vi "niFPGALMRsmpl1MOutSCTL.vi"(0 "input data":fxp<+/-,16,1>, 1 "reset":bool) -> (3 "channel index":u8, 4 "output data":fxp<+/-,18,1> format="%.18g", 10 "output valid":bool)   [LabVIEW 2017]
uses:
  <vilib>/Platform/TimedLoop/XDataNode/timing_clust.ctl
  <vilib>/Platform/TimedLoop/XDataNode/nitl_modes.ctl
  <vilib>/Platform/TimedLoop/XDataNode/wakeup.ctl
  <vilib>/Platform/TimedLoop/XDataNode/XDataNode.xnode
  <vilib>/Platform/TimedLoop/XDataNode/XDNodeRunTimeDep.lvlib
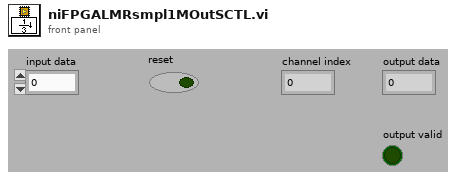
[diagram p1: front panel]
types:
  T1 = typedef "XDNodeRunTimeDep.lvlib/timing_clust.ctl" = cluster{"Expected End [f-1]":u64, "Actual End [f-1]":u64, "Finished Late? [f-1]":bool, "Expected End [i-1]":u64, "Actual End [i-1]":u64, "Finished Late? [i-1]":bool, "Expected Start [i]":u64, "Actual Start [i]":u64, "Expected Start [f]":u64, "Actual Start [f]":u64, "Source Name":string, "Structure Name":string, "Period":i64, "Deadline":i64, "Offset":i64, "Start":i64, "Priority":i32, "Timeout":i32, "Mode":T2, "Wakeup Reason":T3, "Error":errorcluster, "Source Type":string, "Secondary Source Type":string, "Global End Time":u64, "Global Start Time":u64, "Frame Duration":u64, "Iteration Duration":u64, "Assigned CPU":i32, "I/O Scan Engine Mode":u32}
  T2 = typedef "XDNodeRunTimeDep.lvlib/nitl_modes.ctl" = enum32{"No Change", "Process missed periods, maintain original phase", "Discard missed periods, maintain original phase", "Process missed periods, ignore original phase", "Discard missed periods, ignore original phase"}
  T3 = typedef "XDNodeRunTimeDep.lvlib/wakeup.ctl" = enum32{"Normal", "Aborted", "Asynchronous wakeup", "Timing source error", "Timed loop error", "Timeout"}
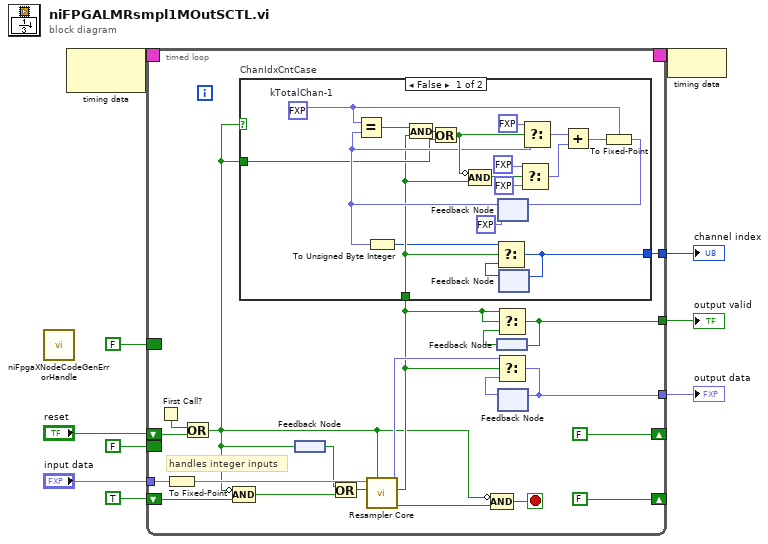
[diagram p0: block diagram]
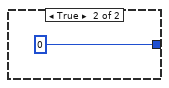
[diagram p2: hidden frame]
diagram:
  n1 = call <vilib>:"niFpgaXNodeCodeGenErrorHandle.vi"() -> ()  [unwired: 1 in]
  n2 = node-c288 ("Input Node")() -> (w8:T1)  [unwired: 1 out]
  n3 = timed-loop "Timed Loop" {
    timing: w8 -> [_]
    timing-out: [_] -> w7
    tunnel: "input data" -> [w27]
    tunnel: [w21] -> w9
    tunnel: [w23] -> w10
    border: FALSE ("dataReady?") -> [_]
    shift-right: [FALSE] -> _
    shift-left: "reset" -> [w17]
    tunnel: [w18] -> w5
    shift-right: [FALSE] -> _
    shift-left: TRUE -> [w25]
    border: FALSE ("reset") -> [_]
    stop <- w22 stop-if-true
    # "handles integer inputs"
    n4 = First Call?() -> (First Call?: T/F=w16:bool)
    n5 = To Fixed-Point(number=w27) -> (fixed-point=w14:fxp<+/-,16,1>)  [unwired: 1 in]
    n6 = Or(x=w16, y=w17) -> (x .or. y?=w11:bool)
    n7 = Compound Arithmetic op=AND(invert w11, w25) -> (w15:bool)
    n8 = feedback-in #1(w11) -> ()
    n9 = feedback #1() -> (w12:bool)
    n10 = Or(x=w12, y=w15) -> (x .or. y?=w13:bool)
    n11 = call "Resampler Core"("reset"=w11, "dataRDYIn"=w13, "datain"=w14) -> ("idle?"=w24:bool, "dataReadyOut"=w19:bool, "output data"=w26:fxp<+/-,18,1>)  [unwired: 6 in]
    n12 = case "ChanIdxCntCase" shown="False" w11 {
      tunnel: w11 -> [w35 _]
      tunnel: [w31 u8 0] -> w18
      tunnel: w19 -> [w34 _]
      frame False {
        w33 = fxp<+,1,1> 0.0  # kTotalChan-1
        n13 = feedback #2(fxp<+,1,1> 0.0) -> (w36:fxp<+,1,1>)
        n14 = Equal?(x=w33, y=w36) -> (x = y?=w47:bool)
        n15 = To Unsigned Byte Integer(number=w36) -> (unsigned 8bit integer=w32:u8)
        n16 = And(x=w47, y=w34) -> (x .and. y?=w46:bool)
        n17 = Or(x=w46, y=w35) -> (x .or. y?=w45:bool)
        n18 = Compound Arithmetic op=AND(invert w45, w34) -> (w42:bool)
        n19 = feedback #3() -> (w49:u8)  [unwired: 1 out]
        n20 = Select(t=w32, s=w34, f=w49) -> (s? t:f=w31:u8)
        n21 = feedback-in #3(w31) -> ()
        n22 = Select(t=fxp<+,1,1> 1.0 ("y"), s=w42, f=fxp<+,1,1> 0.0) -> (s? t:f=w39:fxp<+,1,1>)
        n23 = Select(t=fxp<+,1,1> 0.0 ("y"), s=w45, f=w36) -> (s? t:f=w43:fxp<+,1,1>)
        n24 = Add(x=w43, y=w39) -> (x+y=w38:fxp<+,2,2>)
        n25 = To Fixed-Point(fixed-point type=w33, number=w38) -> (fixed-point=w37:fxp<+,1,1>)
        n26 = feedback-in #2(w37) -> ()
      }
      frame True {
      }
    }
    n27 = Compound Arithmetic op=AND(invert w11, w24) -> (w22:bool)
    n28 = feedback #4() -> (w30:bool)
    n29 = Select(t=w19, s=w19, f=w30) -> (s? t:f=w23:bool)
    n30 = feedback-in #4(w23) -> ()
    n31 = feedback #5() -> (w20:fxp<+/-,18,1>)  [unwired: 1 out]
    n32 = Select(t=w26, s=w19, f=w20) -> (s? t:f=w21:fxp<+/-,18,1>)
    n33 = feedback-in #5(w21) -> ()
  }
  "channel index" <- w5
  "output valid" <- w10
  "output data" <- w9
  n34 = node-c288 ("Output Node")(w7) -> ()
